vi "Open.vi"(8 "error in (no error)":errorcluster, 11 "HAL.TCP in":refnum<class "HAL.TCP.lvclass">) -> (0 "error out":errorcluster, 3 "HAL.TCP out":refnum<class "HAL.TCP.lvclass">)   [LabVIEW 2019, in "HAL.TCP.lvclass"]
uses:
  HAL.TCP.lvclass
  HAL.TCP.lvclass/HAL.TCP.ctl
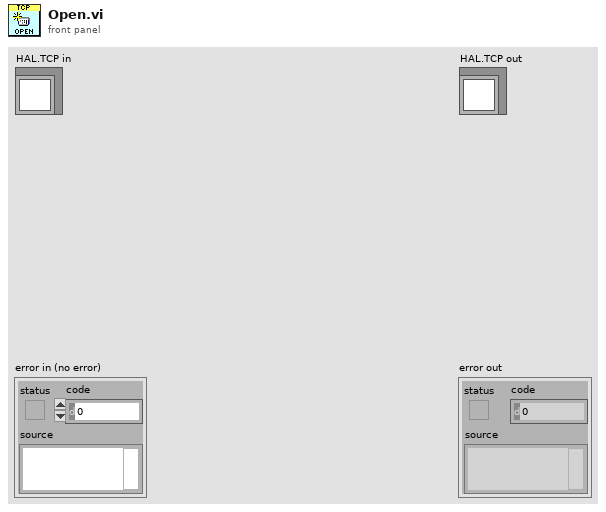
[diagram p1: front panel]
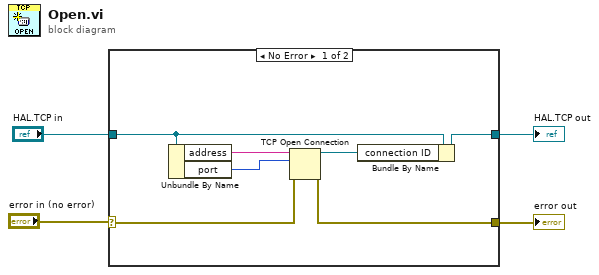
[diagram p0: block diagram]
diagram:
  n1 = case shown="No Error" "error in (no error)" {
    selector: "error in (no error)" -> [w11 w13]
    tunnel: "HAL.TCP in" -> [w10 w12]
    tunnel: [w7 w13] -> w2
    tunnel: [w9 w12] -> w1
    frame No Error {
      n2 = Unbundle By Name(w10) -> ("address"=w6:string, "port"=w5:u16)
      n3 = TCP Open Connection(address=w6, remote port or service name=w5, error in (no error)=w11) -> (connection ID=w8:refnum<k5>, error out=w7:errorcluster)  [unwired: 2 in]
      n4 = Bundle By Name(cluster=w10, "connection ID"=w8) -> (w9:refnum<class "HAL.TCP.lvclass">)
    }
    frame Error {
    }
  }
  "error out" <- w2
  "HAL.TCP out" <- w1
